vi "GV PreframeclockRescanGalvo.vi"() -> ()   [LabVIEW 2017]
panel:
  out "PreframeclockRescanGalvo":bool
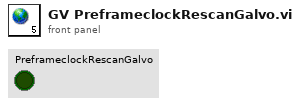
[diagram p1: front panel]
diagram:
